vi "Write_raw_block_header.vi"(1 "No of PWA samples":i32, 2 "Block Timings":T1={"Started"=0.0, "Ended"=0.0, "Analogue Frequency Hz"=1000.0} {"Analogue Frequency Hz" format="%.2f"}, 3 "No of analogue samples":i32, 4 "No of LDA samples":i32) -> (0 "Output string":string)   [LabVIEW 2010]
uses:
  Controls/Block_start_and_end.ctl
  Globals/Meas_global.vi
  Globals/LDA_meas_global_1.vi
  Globals/Plug_in_data_global.vi
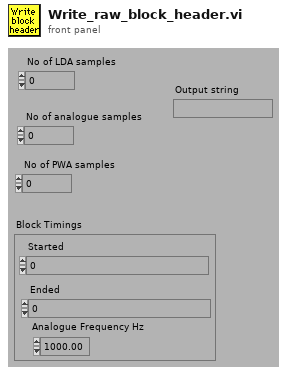
[diagram p1: front panel]
types:
  T1 = typedef "Block_start_and_end.ctl" = cluster{"Started":dbl, "Ended":dbl, "Analogue Frequency Hz":dbl}
  T2 = cluster{"scale multiplier":dbl, "scale offset":dbl}[]
  T3 = typedef "Ch_description_ADAM.ctl" = cluster{"Ch Name":string, "Type":T4, "Function":T5, "Ch State":T6, "Calibration type":T7, "A":dbl, "B":dbl, "C":dbl, "D":dbl, "Comments":string, "Address":T8, "String":string, "Duty":u16}
  T4 = typedef "Module_type_ADAM.ctl" = enum16{"4011", "4012", "4013", "4014", "4016", "4017", "4018", "4021", "4050", "4052", "4053", "4060", "4080", "5000", "5017", "5018", "5024", "5051", "5056", "5060", "6060", "Tracker", "WEST", "GILL", "JEM", "VICI", "Vaisala", "DRUCK", "Run VI Named:", "IR2100", "PPT", "Comparator", "VIRTUAL", "Hold Value", "Read A", "Read Ch", "Coded", "Client Info", "Web Client", "X10", "Test"}
  T5 = typedef "Function_ADAM.ctl" = enum16{"Analogue Input", "Digital Input", "Event counter", "Event rate", "Analogue Output", "Digital Output", "Relay Output"}
  T6 = typedef "Channel_State.ctl" = enum16{"On", "Off", "Always On", "Always Off"}
  T7 = typedef "Calib_type_ADAM.ctl" = enum16{"Raw", "Bx + A", "Cx^2 + Bx + A", "Dx^3 + Cx^2 + Bx + A", "In Band", "Hi-Tec Q", "Hi-Tec M_dot", "Text"}
  T8 = typedef "Address.ctl" = cluster{"Main":i32, "Ch.":i32, "Sub":i32, "Port Name":string}
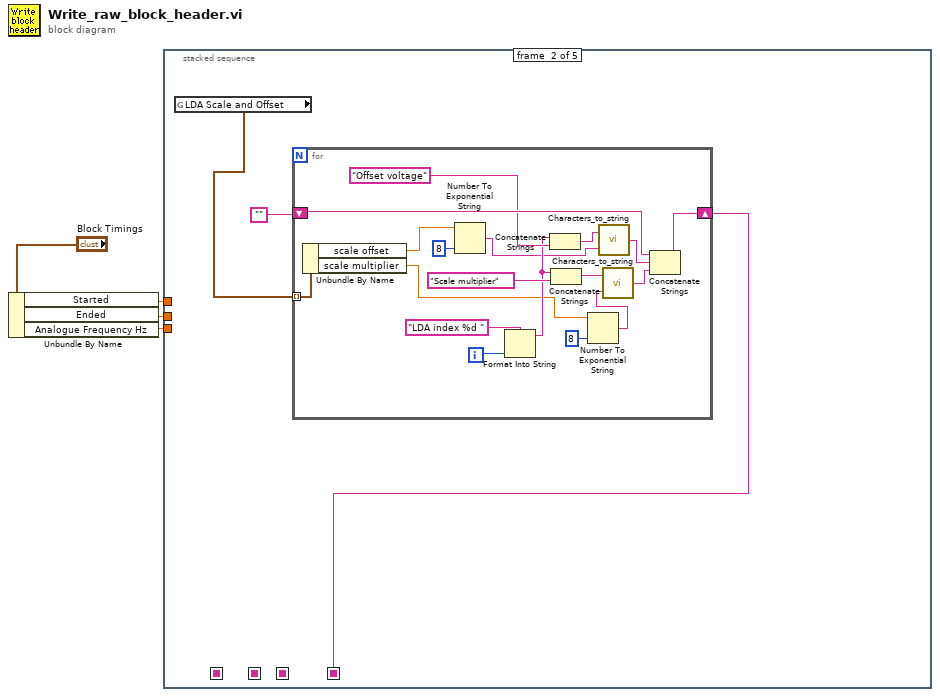
[diagram p0: block diagram]
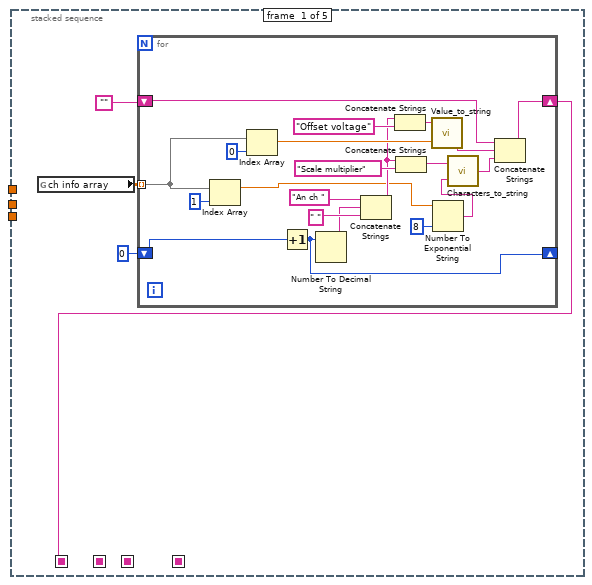
[diagram p2: hidden frame]
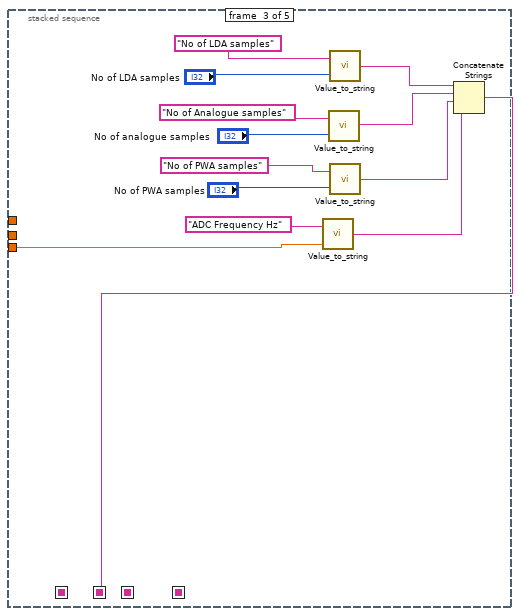
[diagram p3: hidden frame]
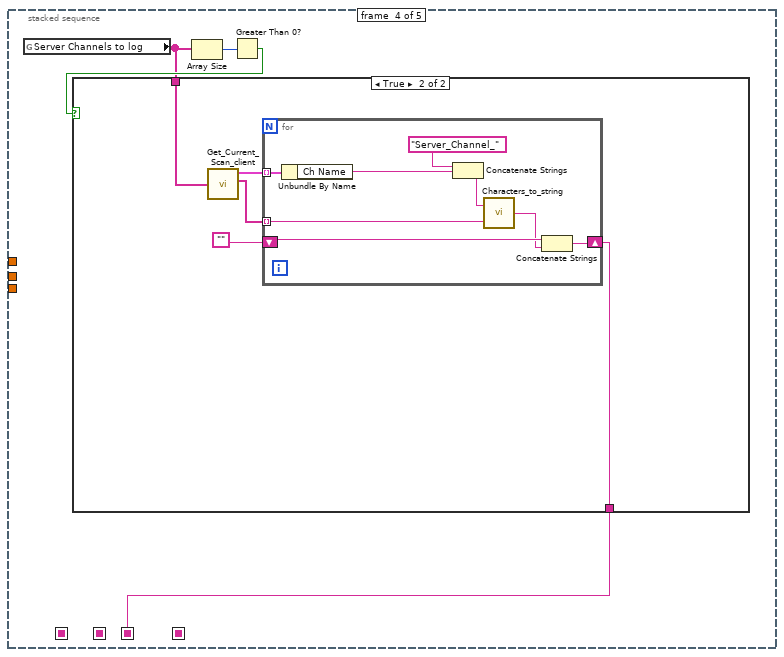
[diagram p4: hidden frame]
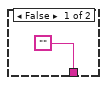
[diagram p5: hidden frame]
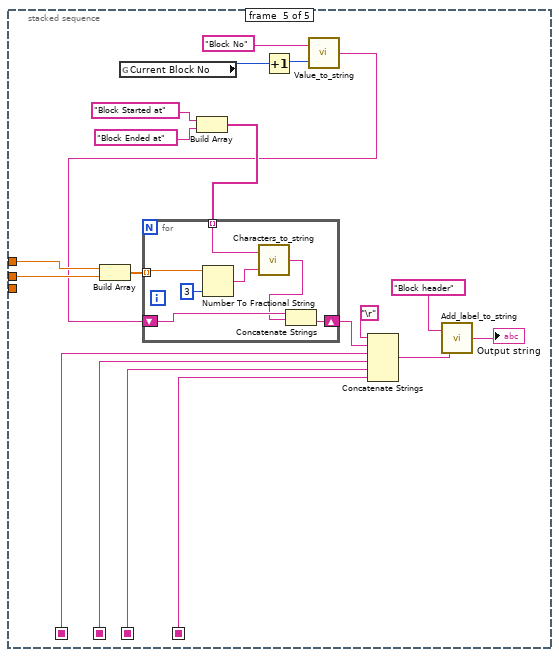
[diagram p6: hidden frame]
diagram:
  n1 = Unbundle By Name("Block Timings") -> ("Started"=w3:dbl, "Ended"=w2:dbl, "Analogue Frequency Hz"=w1:dbl)
  n2 = stacked-sequence {
    seq-local: [w5 _ _ _ _] -> [_ _ _ _ w99]
    seq-local: [_ _ w57 _ _] -> [_ _ _ _ w98]
    seq-local: [_ _ _ w64 _] -> [_ _ _ _ w83]
    seq-local: [_ w30 _ _ _] -> [_ _ _ _ w82]
    tunnel: w3 -> [_ _ _ _ w91]
    tunnel: w2 -> [_ _ _ _ w90]
    tunnel: w1 -> [_ _ w56 _ _]
    frame #0 {
      n3 = global read "Meas_global.vi" "ch info array"() -> (w7:dbl[][])
      n4 = for {
        shift-right: [w28] -> w5
        shift-left: "" -> [w29]
        tunnel: w7 -> [w27] mode=indexing
        shift-right: [w25] -> _
        shift-left: 0 -> [w26]
        n5 = Index Array(array=w27, index=1) -> (element=w9:dbl)
        n6 = Index Array(array=w27, index=0) -> (element=w18:dbl)
        n7 = Increment(x=w26) -> (x+1=w25:i32)
        n8 = Number To Decimal String(number=w25) -> (decimal integer string=w15:string)  [unwired: 1 out]
        n9 = Concatenate Strings("An ch ", w15, " ") -> (w14:string)
        n10 = Concatenate Strings(w14, "Offset voltage") -> (w22:string)
        n11 = Concatenate Strings(w14, "Scale multiplier") -> (w11:string)
        n12 = call "Value_to_string.vi"("Value"=w18, "Label for value"=w22) -> ("Output string"=w24:string)  [unwired: 1 in]
        n13 = Number To Exponential String(number=w9, precision (6)=i16 8) -> (E-format string=w10:string)  [unwired: 2 out]
        n14 = call "Characters_to_string.vi"("Characters to write"=w10, "Label for characters"=w11) -> ("Output string"=w12:string)
        n15 = Concatenate Strings(w29, w24, w12) -> (w28:string)
      }
    }
    frame #1 {
      n16 = global read "LDA_meas_global_1.vi" "LDA Scale and Offset"() -> (w31:T2)
      n17 = for {
        shift-right: [w49] -> w30
        shift-left: "" -> [w50]
        tunnel: w31 -> [w42] mode=indexing
        i -> [w39]
        n18 = Unbundle By Name(w42) -> ("scale offset"=w35:dbl, "scale multiplier"=w38:dbl)
        n19 = Number To Exponential String(number=w35, precision (6)=i16 8) -> (E-format string=w34:string)  [unwired: 2 out]
        n20 = Format Into String(format string="LDA index %d ", w39) -> (resulting string=w40:string)  [unwired: 2 in, 1 out]
        n21 = Concatenate Strings(w40, "Offset voltage") -> (w37:string)
        n22 = Concatenate Strings(w40, "Scale multiplier") -> (w44:string)
        n23 = Number To Exponential String(number=w38, precision (6)=i16 8) -> (E-format string=w43:string)  [unwired: 2 out]
        n24 = call "Characters_to_string.vi"("Characters to write"=w34, "Label for characters"=w37) -> ("Output string"=w33:string)
        n25 = call "Characters_to_string.vi"("Characters to write"=w43, "Label for characters"=w44) -> ("Output string"=w45:string)
        n26 = Concatenate Strings(w50, w33, w45) -> (w49:string)
      }
    }
    frame #2 {
      n27 = call "Value_to_string.vi"("Value"=w56, "Label for value"="ADC Frequency Hz") -> ("Output string"=w51:string)  [unwired: 1 in]
      n28 = call "Value_to_string.vi"("Value"="No of analogue samples", "Label for value"="No of Analogue samples") -> ("Output string"=w58:string)  [unwired: 1 in]
      n29 = call "Value_to_string.vi"("Value"="No of LDA samples", "Label for value"="No of LDA samples") -> ("Output string"=w59:string)  [unwired: 1 in]
      n30 = call "Value_to_string.vi"("Value"="No of PWA samples", "Label for value"="No of PWA samples") -> ("Output string"=w52:string)  [unwired: 1 in]
      n31 = Concatenate Strings(w59, w58, w52, w51) -> (w57:string)
    }
    frame #3 {
      n32 = global read "Plug_in_data_global.vi" "Server Channels to log"() -> (w65:string[])
      n33 = Array Size(array=w65) -> (size(s)=w67:i32)
      n34 = Greater Than 0?(x=w67) -> (x > 0?=w66:bool)
      n35 = case shown="True" w66 {
        tunnel: w65 -> [_ w72]
        tunnel: ["" w69] -> w64
        frame False {
        }
        frame True {
          n36 = call "Get_Current_Scan_client.vi"("ADAM Ch Names"=w72) -> ("Ch Description Array"=w71:T3[], "String values"=w70:string[])  [unwired: 2 out]
          n37 = for {
            shift-right: [w80] -> w69
            shift-left: "" -> [w79]
            tunnel: w71 -> [w76] mode=indexing
            tunnel: w70 -> [w74] mode=indexing
            n38 = Unbundle By Name(w76) -> ("Ch Name"=w75:string)
            n39 = Concatenate Strings("Server_Channel_" ("string"), w75) -> (w77:string)
            n40 = call "Characters_to_string.vi"("Characters to write"=w74, "Label for characters"=w77) -> ("Output string"=w78:string)
            n41 = Concatenate Strings(w79, w78) -> (w80:string)
          }
        }
      }
    }
    frame #4 {
      n42 = Build Array(w91, w90) -> (w92:dbl[])
      n43 = global read "Meas_global.vi" "Current Block No"() -> (w88:i32)
      n44 = Build Array("Block Started at", "Block Ended at") -> (w94:string[])
      n45 = Increment(x=w88) -> (x+1=w84:i32)
      n46 = call "Value_to_string.vi"("Value"=w84, "Label for value"="Block No") -> ("Output string"=w87:string)  [unwired: 1 in]
      n47 = for {
        tunnel: w94 -> [w107] mode=indexing
        shift-right: [w104] -> w96
        shift-left: w87 -> [w106]
        tunnel: w92 -> [w102] mode=indexing
        n48 = Number To Fractional String(number=w102, precision (6)=i16 3) -> (F-format string=w101:string)  [unwired: 2 out]
        n49 = call "Characters_to_string.vi"("Characters to write"=w101, "Label for characters"=w107) -> ("Output string"=w105:string)
        n50 = Concatenate Strings(w106, w105) -> (w104:string)
      }
      n51 = Concatenate Strings("\r", w96, w99, w98, w83, w82) -> (w97:string)
      n52 = call "Add_label_to_string.vi"("String to write"=w97, "File Label"="Block header") -> ("Output string"=→"Output string":string)
    }
  }
